vi "Tosca-Build.vi"() -> ()   [LabVIEW 2020]
uses:
  <vilib>/AppBuilder/AB_API_Simple/Build (path).vi
  <vilib>/AppBuilder/AB_API_Simple/NI_App_Builder_API.lvlib
panel:
  in  "Version":T1={"Major"=4, "Minor"=7, "Fix"=0, "Build"=-1}
  in  "stop":bool
  out "Progress Bar":u8(slide) caption="Finished!" scale=0.0..3.0
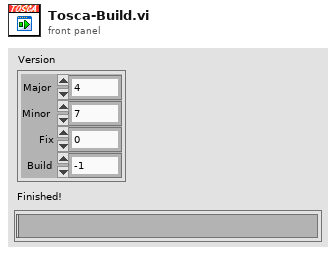
[diagram p1: front panel]
types:
  T1 = cluster{"Major":i32, "Minor":i32, "Fix":i32, "Build":i32}
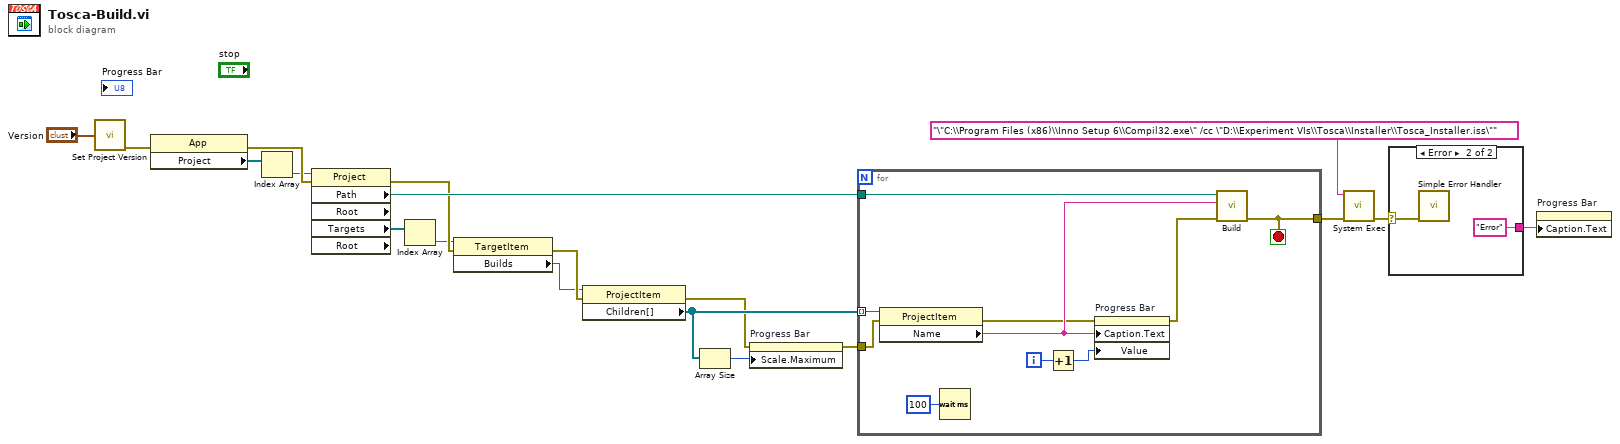
[diagram p0: block diagram]
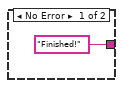
[diagram p2: hidden frame]
diagram:
  n1 = call "Set Project Version.vi"("Version"="Version") -> ("error out"=w1:errorcluster)  [unwired: 14 in]
  n2 = property class="App"(error in=w1) -> (error out=w7:errorcluster, "Project"=w6:refnum<vi>[])  [unwired: 1 in, 1 out]
  n3 = Index Array(array=w6) -> (element=w5:refnum<vi>)  [unwired: 1 in]
  n4 = property class="Project" props=["Path", "Root", "Targets", "Root"](reference=w5, error in=w7) -> (error out=w14:errorcluster, "Path"=w17:path, "Targets"=w4:refnum<vi>[])  [unwired: 3 out]
  n5 = Index Array(array=w4) -> (element=w9:refnum<vi>)  [unwired: 1 in]
  n6 = property class="TargetItem"(reference=w9, error in=w14) -> (error out=w16:errorcluster, "Builds"=w15:refnum<vi>)  [unwired: 1 out]
  n7 = property class="ProjectItem"(reference=w15, error in=w16) -> (error out=w10:errorcluster, "Children[]"=w13:refnum<vi>[])  [unwired: 1 out]
  n8 = Array Size(array=w13) -> (size(s)=w12:i32)
  n9 = property on="Progress Bar" class="Slide (strict)"(error in=w10, "Scale.Maximum"=w12) -> (error out=w11:errorcluster)  [unwired: 1 in, 1 out]
  n10 = for {
    tunnel: w17 -> [w29]
    tunnel: w13 -> [w28] mode=indexing
    tunnel: [w24] -> w3
    tunnel: w11 -> [w23]
    i -> [w27]
    stop <- w24 stop-if-true
    n11 = property class="ProjectItem"(reference=w28, error in=w23) -> (error out=w21:errorcluster, "Name"=w22:string)  [unwired: 1 out]
    n12 = Wait (ms)(milliseconds to wait=u32 100) -> ()  [unwired: 1 out]
    n13 = Increment(x=w27) -> (x+1=w26:i32)
    n14 = property on="Progress Bar" class="Slide (strict)"(error in=w21, "Caption.Text"=w22, "Value"=w26) -> (error out=w20:errorcluster)  [unwired: 1 in, 1 out]
    n15 = call-poly <vilib>:"Build.vi"("error in (no error)"=w20, "Name of build specification (if empty: build all)"=w22, "Path to project"=w29) -> ("error out"=w24:errorcluster)  [unwired: 7 in, 1 out]
  }
  n16 = call <vilib>:"System Exec.vi"("error in (no error)"=w3, "command line"="\"C:\\Program Files (x86)\\Inno Setup 6\\Compil32.exe\" /cc \"D:\\Experiment VIs\\Tosca\\Installer\\Tosca_Installer.iss\"") -> ("error out"=w18:errorcluster)  [unwired: 6 in, 3 out]
  n17 = case shown="Error" w18 {
    selector: w18 -> [_ w31]
    tunnel: ["Finished!" "Error"] -> w19
    frame No Error {
    }
    frame Error {
      n18 = call <vilib>:"Simple Error Handler.vi"("error in (no error)"=w31) -> ()  [unwired: 4 in, 5 out]
    }
  }
  n19 = property on="Progress Bar" class="Slide (strict)"("Caption.Text"=w19) -> ()  [unwired: 2 in, 2 out]
